vi "evo irimager terminate.vi"() -> (3 "function return":i32)   [LabVIEW 2017, in "libirimager_direct_binding.lvlib"]
doc: "DIRECT_API int evo_irimager_terminate();"
uses:
  libirimager_direct_binding.lvlib
  labview/libirimager.dll
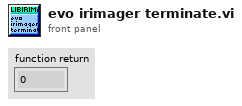
[diagram p1: front panel]
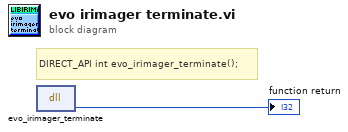
[diagram p0: block diagram]
diagram:
  # "DIRECT_API int evo_irimager_terminate();"
  n1 = dll-call lib="C:/Users/HelmutEngelhardt/Documents/labview/libirimager.dll" fn="evo_irimager_terminate"() -> ("Rückgabetyp"=→"function return":i32)  [unwired: 3 in, 2 out]
